vi "TestObserveError_ValueTrueCode1.vi"(8 "error in (no error)":errorcluster, 11 "TestCase in":refnum<class "TestObservableDataTypes.lvclass">) -> (0 "error out":errorcluster, 3 "TestCase out":refnum<class "TestObservableDataTypes.lvclass">)   [LabVIEW 2017, in "TestObservableDataTypes.lvclass"]
uses:
  TestObservableDataTypes.lvclass
  Source/Framework/IMediator/IMediator Messages/Subscribe Msg/Subscribe Msg.lvclass
  Source/Framework/IMediator/SubscriptionRequest/SubscriptionRequest.lvclass
  Source/Framework/IMediator/ISubscriptionPolicy/ISubscriptionPolicy.lvclass
  Source/Framework/SubscriptionPolicy/BasicSubscription/BasicSubscription.lvclass
  C:/Git/mva-framework/Source/Framework/IMediator/ISubscriptionPolicy/ISubscriptionPolicy.lvclass
  gpm_packages/@cs/transport/Source/ITransport/ITransport.lvclass
panel:
  out "ControlTerminal":errorcluster
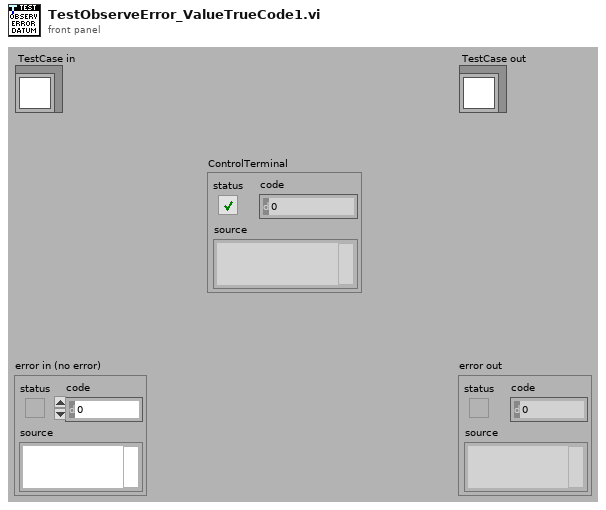
[diagram p1: front panel]
types:
  T1 = typedef "IMediator.lvlib/ISubscriptionPolicy.lvclass/ISubscriptionPolicy Reference.ctl" = refnum<data-value>
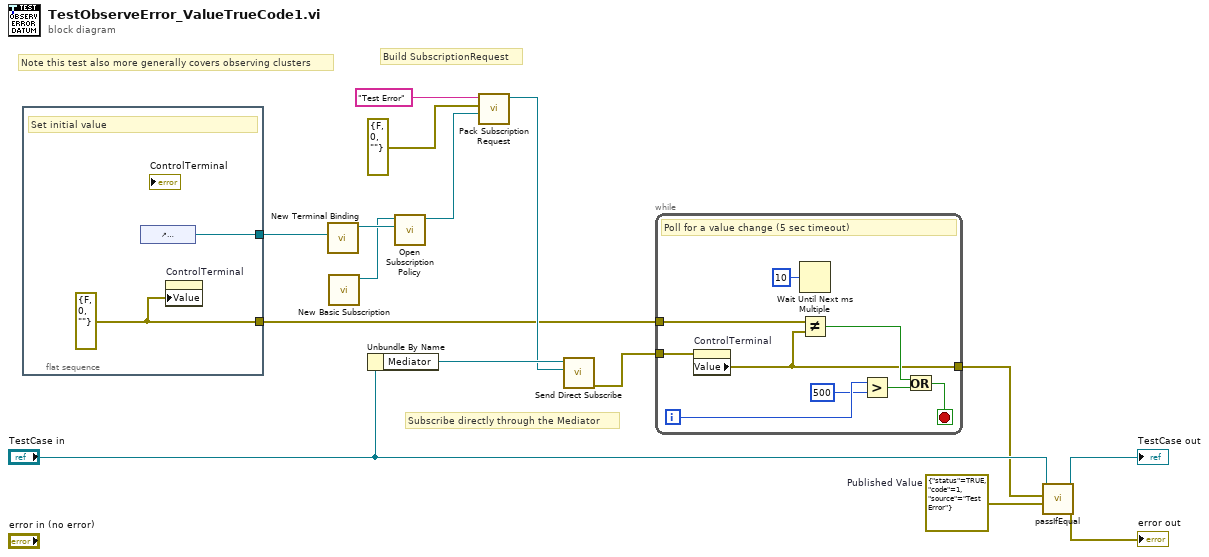
[diagram p0: block diagram]
diagram:
  w3 = errorcluster {"status"=TRUE, "code"=1, "source"="Test Error"}  # Published Value
  # "Note this test also more generally covers observing clusters"
  # "Build SubscriptionRequest"
  # "Subscribe directly through the Mediator"
  n1 = flat-sequence {
    tunnel: [w17] -> w7
    tunnel: [w16] -> w5
    frame #0 {
      w16 = errorcluster {"status"=FALSE, "code"=0, "source"=""} ("ControlTerminal")
      # "Set initial value"
      n2 = control-ref of="ControlTerminal"() -> (w17:refnum<vi>)
      n3 = property on="ControlTerminal" class="Clust (strict)"("Value"=w16) -> ()  [unwired: 2 in, 2 out]
    }
  }
  n4 = call "New Terminal Binding.vi"("Ctl Refnum"=w7) -> ("TerminalBinding"=w8:refnum<class "TerminalBinding.lvclass">)  [unwired: 9 in, 1 out]
  n5 = call "New Basic Subscription.vi"() -> ("BasicSubscription Out"=w2:refnum<class "BasicSubscription.lvclass">)  [unwired: 11 in]
  n6 = Unbundle By Name("TestCase in") -> ("Mediator"=w12:refnum<class "Message Enqueuer.lvclass">)
  n7 = call "Open Subscription Policy.vi"("Transport"=w8, "SubscriptionPolicy"=w2) -> ("Subscription Policy"=w1:T1)  [unwired: 8 in, 1 out]
  n8 = call "Pack Subscription Request.vi"("Subscription Policy"=w1, "Type"=errorcluster {"status"=FALSE, "code"=0, "source"=""}, "Datum Name"="Test Error" ("Topic Name")) -> ("SubscriptionRequest"=w11:refnum<class "SubscriptionRequest.lvclass">)  [unwired: 8 in]
  n9 = call "Send Direct Subscribe.vi"("Subscription Request"=w11, "Message Enqueuer"=w12) -> ("error out"=w6:errorcluster)  [unwired: 8 in, 1 out]
  n10 = while {
    tunnel: w6 -> [w26]
    tunnel: w5 -> [w25]
    tunnel: [w18] -> w4
    i -> [w21]
    stop <- w19 stop-if-true
    # "Poll for a value change (5 sec timeout)"
    n11 = property on="ControlTerminal" class="Clust (strict)"(error in=w26) -> ("Value"=w18:errorcluster)  [unwired: 1 in, 2 out]
    n12 = Wait Until Next ms Multiple(millisecond multiple=u32 10 ("milliseconds to wait")) -> ()  [unwired: 1 out]
    n13 = Not Equal?(x=w25, y=w18) -> (x != y?=w24:bool)
    n14 = Greater?(x=w21, y=500) -> (0:w22:bool)
    n15 = Or(x=w24, y=w22) -> (x .or. y?=w19:bool)
  }
  n16 = call-dynamic "passIfEqual.vi"("y"=w3, "x"=w4, "TestCase in"="TestCase in") -> ("error out"=→"error out":errorcluster, "TestCase out"=→"TestCase out":refnum<class "TestObservableDataTypes.lvclass">)  [unwired: 7 in]
